vi "conditionally close vi ref.vi"(7 "new ref?":bool, 8 "error in (no error)":errorcluster, 11 "vi ref":refnum<vi>) -> (0 "error out":errorcluster)   [LabVIEW 2024, in "controls manager.lvlib"]
uses:
  controls manager.lvlib
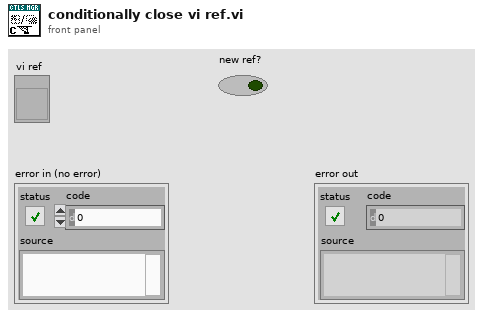
[diagram p1: front panel]
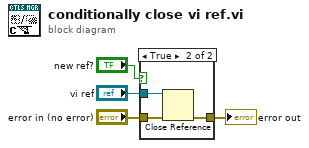
[diagram p0: block diagram]
diagram:
  n1 = case shown="True" "new ref?" {
    tunnel: "error in (no error)" -> [w5 w8]
    tunnel: [w5 w7] -> w2
    tunnel: "vi ref" -> [_ w6]
    frame False {
    }
    frame True {
      n2 = Close Reference(reference=w6, error in (no error)=w8) -> (error out=w7:errorcluster)
    }
  }
  "error out" <- w2
